vi "Query Dig.vi"() -> ()   [LabVIEW 2016, in "数据传输系统-06.lvlib"]
panel:
  out "水深":string[][](array[string])
  in  "Combo Box":string(combo)
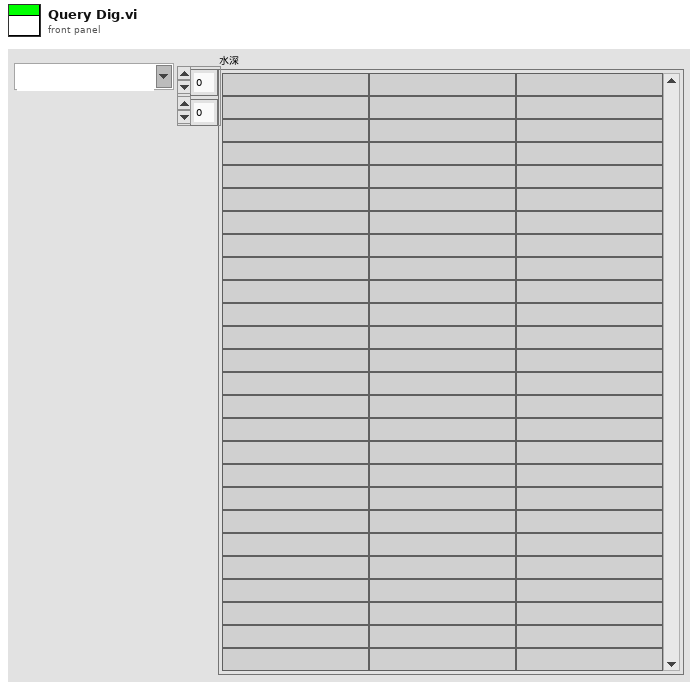
[diagram p1: front panel]
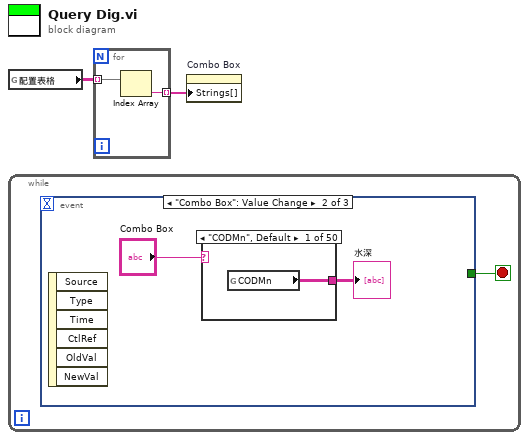
[diagram p0: block diagram]
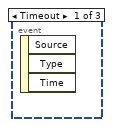
[diagram p2: hidden frame]
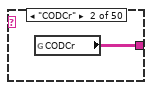
[diagram p3: hidden frame]
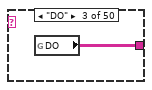
[diagram p4: hidden frame]
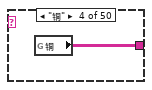
[diagram p5: hidden frame]
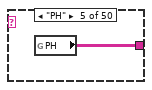
[diagram p6: hidden frame]
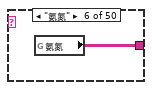
[diagram p7: hidden frame]
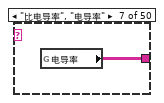
[diagram p8: hidden frame]
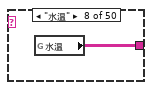
[diagram p9: hidden frame]
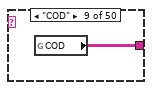
[diagram p10: hidden frame]
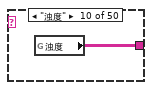
[diagram p11: hidden frame]
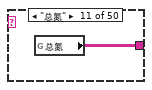
[diagram p12: hidden frame]
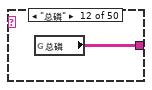
[diagram p13: hidden frame]
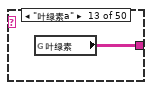
[diagram p14: hidden frame]
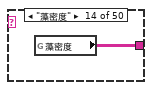
[diagram p15: hidden frame]
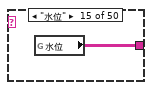
[diagram p16: hidden frame]
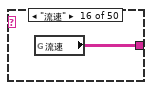
[diagram p17: hidden frame]
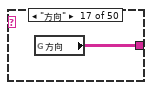
[diagram p18: hidden frame]
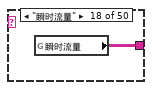
[diagram p19: hidden frame]
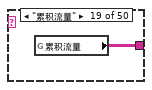
[diagram p20: hidden frame]
diagram:
  n1 = global read "断电保存全局.vi" "配置表格"() -> (w2:string[][])
  n2 = while {
    stop <- w3 stop-if-true
    n3 = event shown="[1] \"Combo Box\": Value Change" {
      selector: _ -> [_ _ _]
      dyn-events: _ -> [_ _ _]
      timeout: _ -> [_ _ _]
      tunnel: [_ _ TRUE] -> w3
      event Timeout {
        n4 = event-data() -> ()  [unwired: 1 in, 3 out]
      }
      event "Combo Box": Value Change {
        n5 = event-data() -> ()  [unwired: 1 in, 6 out]
        n6 = case shown="\"CODMn\", Default" "Combo Box" {
          tunnel: [w6 w7 w8 w9 w10 w11 w12 w13 w14 w15 w16 w17 w18 w19 w20 w21 w22 w23 w24 w25 w26 w27 w28 w29 w30 w31 w32 w33 w34 w35 w36 w37 w38 w39 w40 w41 w42 w43 w44 w45 w46 w47 w48 w49 w50 w51 w52 w53 w54 w55] -> w5
          frame "CODMn", Default {
            n7 = global read "全局 所有参数.vi" "CODMn"() -> (w6:string[][])
          }
          frame "CODCr" {
            n8 = global read "全局 所有参数.vi" "CODCr"() -> (w7:string[][])
          }
          frame "DO" {
            n9 = global read "全局 所有参数.vi" "DO"() -> (w8:string[][])
          }
          frame "铜" {
            n10 = global read "全局 所有参数.vi" "铜"() -> (w9:string[][])
          }
          frame "PH" {
            n11 = global read "全局 所有参数.vi" "PH"() -> (w10:string[][])
          }
          frame "氨氮" {
            n12 = global read "全局 所有参数.vi" "氨氮"() -> (w11:string[][])
          }
          frame "比电导率", "电导率" {
            n13 = global read "全局 所有参数.vi" "电导率"() -> (w12:string[][])
          }
          frame "水温" {
            n14 = global read "全局 所有参数.vi" "水温"() -> (w13:string[][])
          }
          frame "COD" {
            n15 = global read "全局 所有参数.vi" "COD"() -> (w14:string[][])
          }
          frame "浊度" {
            n16 = global read "全局 所有参数.vi" "浊度"() -> (w15:string[][])
          }
          frame "总氮" {
            n17 = global read "全局 所有参数.vi" "总氮"() -> (w16:string[][])
          }
          frame "总磷" {
            n18 = global read "全局 所有参数.vi" "总磷"() -> (w17:string[][])
          }
          frame "叶绿素a" {
            n19 = global read "全局 所有参数.vi" "叶绿素"() -> (w18:string[][])
          }
          frame "藻密度" {
            n20 = global read "全局 所有参数.vi" "藻密度"() -> (w19:string[][])
          }
          frame "水位" {
            n21 = global read "全局 所有参数.vi" "水位"() -> (w20:string[][])
          }
          frame "流速" {
            n22 = global read "全局 所有参数.vi" "流速"() -> (w21:string[][])
          }
          frame "方向" {
            n23 = global read "全局 所有参数.vi" "方向"() -> (w22:string[][])
          }
          frame "瞬时流量" {
            n24 = global read "全局 所有参数.vi" "瞬时流量"() -> (w23:string[][])
          }
          frame "累积流量" {
            n25 = global read "全局 所有参数.vi" "累积流量"() -> (w24:string[][])
          }
          frame "正累积流量" {
            n26 = global read "全局 所有参数.vi" "正累积流量"() -> (w25:string[][])
          }
          frame "负累积流量" {
            n27 = global read "全局 所有参数.vi" "负累积流量"() -> (w26:string[][])
          }
          frame "亚硝氮" {
            n28 = global read "全局 所有参数.vi" "亚硝酸盐"() -> (w27:string[][])
          }
          frame "硫化物" {
            n29 = global read "全局 所有参数.vi" "硫化物"() -> (w28:string[][])
          }
          frame "ORP" {
            n30 = global read "全局 所有参数.vi" "ORP"() -> (w29:string[][])
          }
          frame "铅" {
            n31 = global read "全局 所有参数.vi" "铅"() -> (w30:string[][])
          }
          frame "镉" {
            n32 = global read "全局 所有参数.vi" "镉"() -> (w31:string[][])
          }
          frame "锌" {
            n33 = global read "全局 所有参数.vi" "锌"() -> (w32:string[][])
          }
          frame "镍" {
            n34 = global read "全局 所有参数.vi" "镍"() -> (w33:string[][])
          }
          frame "锰" {
            n35 = global read "全局 所有参数.vi" "锰"() -> (w34:string[][])
          }
          frame "汞" {
            n36 = global read "全局 所有参数.vi" "汞"() -> (w35:string[][])
          }
          frame "气温" {
            n37 = global read "全局 所有参数.vi" "气温"() -> (w36:string[][])
          }
          frame "气压" {
            n38 = global read "全局 所有参数.vi" "气压"() -> (w37:string[][])
          }
          frame "风速" {
            n39 = global read "全局 所有参数.vi" "风速"() -> (w38:string[][])
          }
          frame "风向" {
            n40 = global read "全局 所有参数.vi" "风向"() -> (w39:string[][])
          }
          frame "空气温度" {
            n41 = global read "全局 所有参数.vi" "空气温度"() -> (w40:string[][])
          }
          frame "相对湿度" {
            n42 = global read "全局 所有参数.vi" "相对湿度"() -> (w41:string[][])
          }
          frame "分钟雨量" {
            n43 = global read "全局 所有参数.vi" "分钟雨量"() -> (w42:string[][])
          }
          frame "小时雨量" {
            n44 = global read "全局 所有参数.vi" "小时雨量"() -> (w43:string[][])
          }
          frame "日雨量" {
            n45 = global read "全局 所有参数.vi" "日雨量"() -> (w44:string[][])
          }
          frame "累积雨量" {
            n46 = global read "全局 所有参数.vi" "累积雨量"() -> (w45:string[][])
          }
          frame "盐度" {
            n47 = global read "全局 所有参数.vi" "盐度"() -> (w46:string[][])
          }
          frame "磷酸盐" {
            n48 = global read "全局 所有参数.vi" "磷酸盐"() -> (w47:string[][])
          }
          frame "硝氮" {
            n49 = global read "全局 所有参数.vi" "硝氮"() -> (w48:string[][])
          }
          frame "氟化物" {
            n50 = global read "全局 所有参数.vi" "氟化物"() -> (w49:string[][])
          }
          frame "挥发酚" {
            n51 = global read "全局 所有参数.vi" "挥发酚"() -> (w50:string[][])
          }
          frame "氯化物" {
            n52 = global read "全局 所有参数.vi" "氯化物"() -> (w51:string[][])
          }
          frame "蓝绿藻" {
            n53 = global read "全局 所有参数.vi" "蓝绿藻"() -> (w52:string[][])
          }
          frame "余氯" {
            n54 = global read "全局 所有参数.vi" "余氯"() -> (w53:string[][])
          }
          frame "综合生物毒性" {
            n55 = global read "全局 所有参数.vi" "综合生物毒性"() -> (w54:string[][])
          }
          frame "水深" {
            n56 = global read "全局 所有参数.vi" "水深"() -> (w55:string[][])
          }
        }
        "水深" <- w5
      }
      event Panel Close? {
        n57 = event-data() -> ()  [unwired: 1 in, 4 out]
        n58 = event-data("Discard?"=TRUE) -> ()  [unwired: 1 in, 1 out]
      }
    }
  }
  n59 = for {
    tunnel: w2 -> [w59] mode=indexing
    tunnel: [w58] -> w1 mode=indexing
    n60 = Index Array(array=w59) -> (element=w58:string)  [unwired: 1 in]
  }
  n61 = property on="Combo Box" class="CmbBox"("Strings[]"=w1) -> ()  [unwired: 2 in, 2 out]
